vi "Initialize.vi"(8 "error in (no error)":errorcluster caption="Fehler (Eingang, kein Fehler)", 10 "Baud Rate":u16(ring)=4 items=["300", "1200", "2400", "4800", "9600", "19200", "38400"], 11 "input refnum":refnum<visa-resource-name> caption="Eingang (Referenz)") -> (0 "Cluster (Ausgang)":errorcluster, 3 "Referenz out":refnum<visa-resource-name>)   [LabVIEW 2017, in "Dual Gauge.lvlib"]
uses:
  <userlib>/Dual Gauge/Dual Gauge.lvlib
panel:
  out "Def. Value":u16=3
  in  "Max Value":u16=5
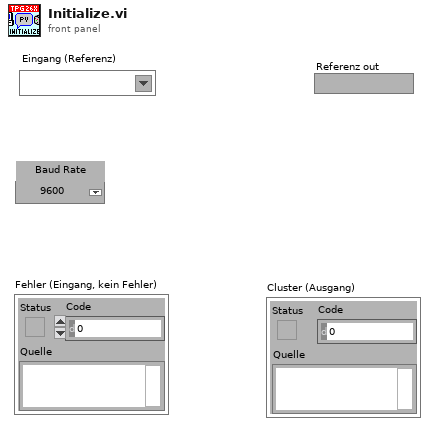
[diagram p1: front panel]
types:
  T1 = enum16{"Init & Test", "Next Baud Rate", "Set Default ", "Communication OK", "Error Box"}
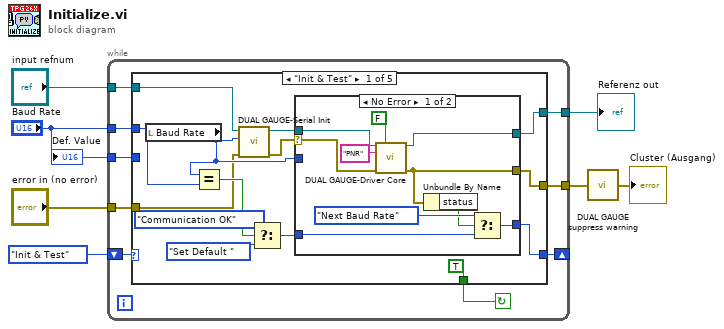
[diagram p0: block diagram]
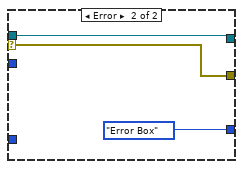
[diagram p2: hidden frame]
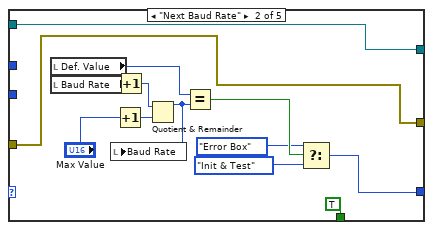
[diagram p3: hidden frame]
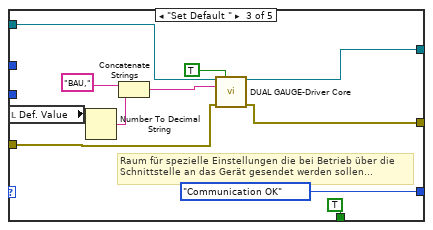
[diagram p4: hidden frame]
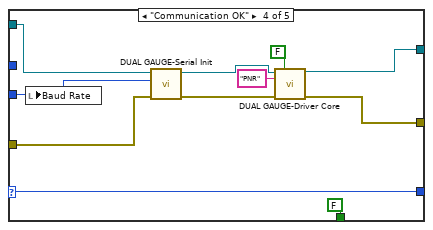
[diagram p5: hidden frame]
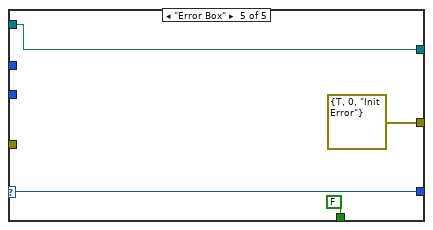
[diagram p6: hidden frame]
diagram:
  n1 = while {
    tunnel: "Baud Rate" -> [w12]
    tunnel: "Baud Rate" -> [w16]
    shift-left: T1."Init & Test" -> [w15]
    shift-right: [w13] -> _
    tunnel: "input refnum" -> [w11]
    tunnel: "error in (no error)" -> [w10]
    tunnel: [w9] -> w2
    tunnel: [w8] -> w3
    stop <- w14 continue-if-true
    n2 = case shown="\"Init & Test\"" w15 {
      selector: w15 -> [_ _ _ w77 w81]
      tunnel: w16 -> [w29 _ _ _ _]
      tunnel: [TRUE TRUE TRUE FALSE FALSE] -> w14
      tunnel: [w24 w47 T1."Communication OK" w77 w81] -> w13
      tunnel: w12 -> [_ _ _ w75 _]
      tunnel: w11 -> [w21 w45 w60 w74 w79]
      tunnel: w10 -> [w19 w44 w59 w72 _]
      tunnel: [w17 w44 w57 w71 errorcluster {"status"=TRUE, "code"=0, "source"="Init Error"} ("Cluster (Ausgang)")] -> w9
      tunnel: [w18 w45 w58 w70 w79] -> w8
      frame "Init & Test" {
        n3 = local read "Baud Rate"() -> (w22:u16)
        n4 = Equal?(x=w22, y=w29) -> (x = y?=w28:bool)
        n5 = call <userlib>:"DUAL GAUGE-Serial Init.vi"("error in (no error)"=w19, "Baud Rate"=w22, "input refnum"=w21) -> ("error out"=w30:errorcluster, "VISA resource out"=w20:refnum<visa-resource-name>)  [unwired: 7 in]
        n6 = Select(t=T1."Communication OK", s=w28, f=T1."Set Default ") -> (s? t:f=w27:T1)
        n7 = case shown="No Error" w30 {
          selector: w30 -> [w34 w41]
          tunnel: [w40 T1."Error Box"] -> w24
          tunnel: w27 -> [w38 _]
          tunnel: w22 -> [_ _]
          tunnel: w20 -> [w35 w42]
          tunnel: [w33 w42] -> w18
          tunnel: [w31 w41] -> w17
          frame No Error {
            n8 = call <userlib>:"DUAL GAUGE-Driver Core.vi"("Referenz in"=w35, "Write/Read"=FALSE, "Command"="PNR", "Fehler (Eingang)"=w34) -> ("Referenz out"=w33:refnum<visa-resource-name>, "Cluster (Ausgang)"=w31:errorcluster)  [unwired: 9 in, 1 out]
            n9 = Unbundle By Name(w31) -> ("status"=w32:bool)
            n10 = Select(t=T1."Next Baud Rate", s=w32, f=w38) -> (s? t:f=w40:T1)
          }
          frame Error {
          }
        }
      }
      frame "Next Baud Rate" {
        n11 = local read "Def. Value"() -> (w53:u16)
        n12 = local read "Baud Rate"() -> (w46:u16)
        n13 = Increment(x="Max Value") -> (x+1=w54:u16)
        n14 = Increment(x=w46) -> (x+1=w56:u16)
        n15 = Quotient & Remainder(x=w56, y=w54) -> (x-y*floor(x/y)=w52:u16)  [unwired: 1 out]
        n16 = local write "Baud Rate"(w52) -> ()
        n17 = Equal?(x=w53, y=w52) -> (x = y?=w51:bool)
        n18 = Select(t=T1."Error Box", s=w51, f=T1."Init & Test") -> (s? t:f=w47:T1)
      }
      frame "Set Default " {
        # "Raum für spezielle Einstellungen die bei Betrieb über die\nSchnittstelle an das Gerät gesendet werden sollen..."
        n19 = local read "Def. Value"() -> (w63:u16)
        n20 = Number To Decimal String(number=w63) -> (decimal integer string=w62:string)  [unwired: 1 in]
        n21 = Concatenate Strings("BAU,", w62) -> (w61:string)
        n22 = call <userlib>:"DUAL GAUGE-Driver Core.vi"("Referenz in"=w60, "Write/Read"=TRUE, "Command"=w61, "Fehler (Eingang)"=w59) -> ("Referenz out"=w58:refnum<visa-resource-name>, "Cluster (Ausgang)"=w57:errorcluster)  [unwired: 9 in, 1 out]
      }
      frame "Communication OK" {
        n23 = local write "Baud Rate"(w75) -> ()
        n24 = call <userlib>:"DUAL GAUGE-Serial Init.vi"("error in (no error)"=w72, "Baud Rate"=w75, "input refnum"=w74) -> ("error out"=w76:errorcluster, "VISA resource out"=w73:refnum<visa-resource-name>)  [unwired: 7 in]
        n25 = call <userlib>:"DUAL GAUGE-Driver Core.vi"("Referenz in"=w73, "Write/Read"=FALSE, "Command"="PNR", "Fehler (Eingang)"=w76) -> ("Referenz out"=w70:refnum<visa-resource-name>, "Cluster (Ausgang)"=w71:errorcluster)  [unwired: 9 in, 1 out]
      }
      frame "Error Box" {
      }
    }
  }
  "Referenz out" <- w3
  n26 = call <userlib>:"DUAL GAUGE suppress warning.vi"("error in"=w2) -> ("error out"=→"Cluster (Ausgang)":errorcluster)
  "Def. Value" <- "Baud Rate"
